vi "ReadConfigFile.vi"(1 "ConfigFilePath":path) -> (0 "Inst_parameters":T1)   [LabVIEW 2013]
uses:
  <vilib>/addons/h5labview2/file/H5Fmode.ctl
  <vilib>/addons/h5labview2/base/lib_path.vi
  <vilib>/addons/h5labview2/base/H5Equery.vi
  <vilib>/addons/h5labview2/attrib/H5Aread.llb/H5Aread.xnode
  <vilib>/addons/h5labview2/base/hid_t.ctl
  <vilib>/addons/h5labview2/file/H5F.lvlib
panel:
  out "Inst_list":string[](array[string])
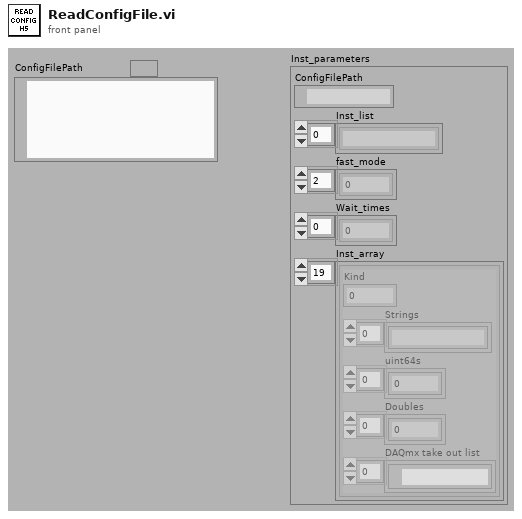
[diagram p1: front panel]
types:
  T1 = cluster{"ConfigFilePath":path, "Inst_list":string[], "fast_mode":u64[], "Wait_times":u64[], "Inst_array":cluster{"Kind":u16, "Strings":string[], "uint64s":u64[], "Doubles":dbl[], "DAQmx take out list":refnum<k21>[]}[]}
  T2 = cluster{"ConfigFilePath":path, "Inst_list":string[], "fast_mode":u16[], "Wait_times":u64[], "Inst_array":cluster{"Kind":u16, "Strings":string[], "uint16s":u64[], "Doubles":dbl[], refnum<k21>[]}[]}
  T3 = typedef "H5F.lvlib/H5Fmode.ctl" = enum16{"read-only", "read-write", "overwrite", "create new", "open or create"}
  T4 = cluster{"Kind":u16, "Strings":string[], "uint16s":u64[], "Doubles":dbl[], refnum<k21>[]}
  T5 = typedef "hid_t.ctl" = i32
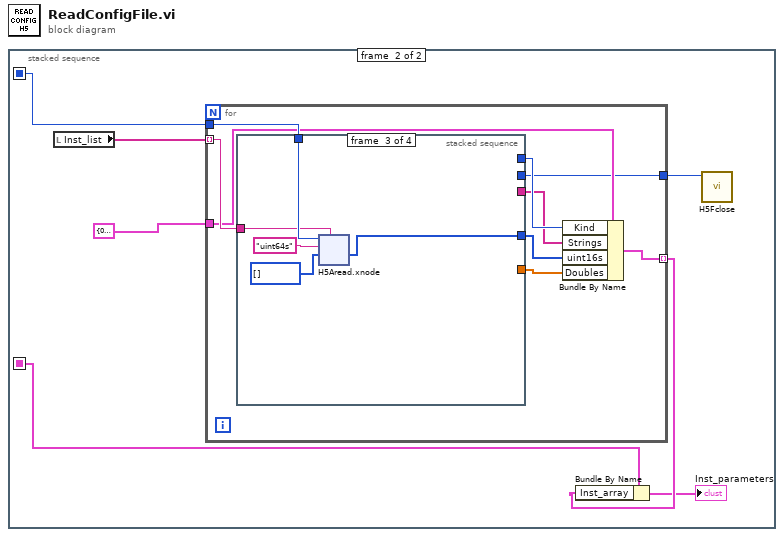
[diagram p0: block diagram]
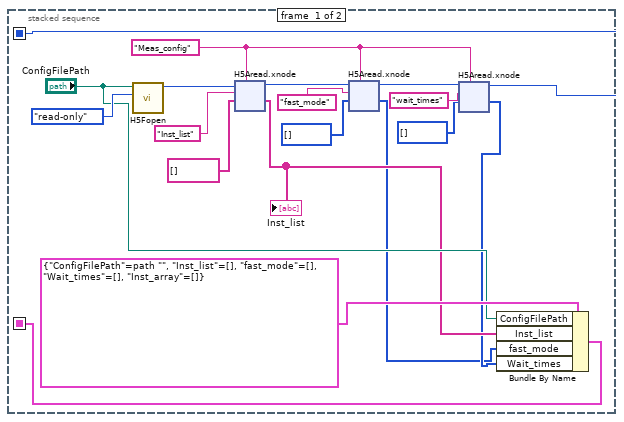
[diagram p2: hidden frame]
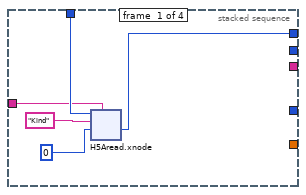
[diagram p3: hidden frame]
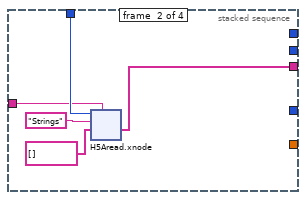
[diagram p4: hidden frame]
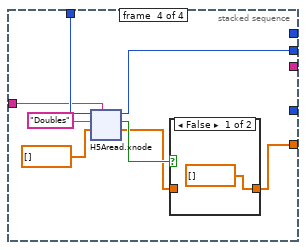
[diagram p5: hidden frame]
diagram:
  n1 = stacked-sequence {
    seq-local: [w1 _] -> [_ w69]
    seq-local: [w3 _] -> [_ w66]
    frame #0 {
      w9 = "Meas_config"
      n2 = call <vilib>:"H5Fopen.vi"("mode (read-only)"=H5Fmode."read-only" ("mode"), "path"="ConfigFilePath") -> ("ref out"=w16:T5)  [unwired: 8 in, 1 out]
      n3 = xnode "H5Aread.xnode"("object name"=w9, "default"=string[] [], "attrib name"="Inst_list", "ref in"=w16) -> ("data"=w5:string[], "ref out"=w14:T5)  [unwired: 2 in, 2 out]
      "Inst_list" <- w5
      n4 = xnode "H5Aread.xnode"("object name"=w9, "default"=u16[] [], "attrib name"="fast_mode", "ref in"=w14) -> ("data"=w2:u16[], "ref out"=w12:T5)  [unwired: 2 in, 2 out]
      n5 = xnode "H5Aread.xnode"("object name"=w9, "default"=u64[] [], "attrib name"="wait_times", "ref in"=w12) -> ("data"=w4:u64[], "ref out"=w1:T5)  [unwired: 2 in, 2 out]
      n6 = Bundle By Name(cluster=T2 {"ConfigFilePath"=path "", "Inst_list"=[], "fast_mode"=[], "Wait_times"=[], "Inst_array"=[]}, "ConfigFilePath"="ConfigFilePath", "Inst_list"=w5, "fast_mode"=w2, "Wait_times"=w4) -> (w3:T2)
    }
    frame #1 {
      n7 = local read "Inst_list"() -> (w70:string[])
      n8 = for {
        tunnel: w70 -> [w79] mode=indexing
        tunnel: w69 -> [w78]
        tunnel: T4 {"Kind"=0, "Strings"=[], "uint16s"=[], "Doubles"=[], []} -> [w76]
        tunnel: [w72] -> w65 mode=indexing
        tunnel: [w71] -> w67
        n9 = stacked-sequence {
          tunnel: w79 -> [w80 w100 w120 w140]
          tunnel: w78 -> [w83 w103 w123 w146]
          tunnel: [w81 _ _ _] -> w77
          tunnel: [_ w101 _ _] -> w75
          tunnel: [_ _ w121 _] -> w74
          tunnel: [_ _ _ w142] -> w73
          tunnel: [_ _ _ w141] -> w71
          frame #0 {
            n10 = xnode "H5Aread.xnode"("object name"=w80, "default"=u16 0, "attrib name"="Kind", "ref in"=w83) -> ("data"=w81:u16)  [unwired: 2 in, 3 out]
          }
          frame #1 {
            n11 = xnode "H5Aread.xnode"("object name"=w100, "default"=string[] [], "attrib name"="Strings", "ref in"=w103) -> ("data"=w101:string[])  [unwired: 2 in, 3 out]
          }
          frame #2 {
            n12 = xnode "H5Aread.xnode"("object name"=w120, "default"=u64[] [], "attrib name"="uint64s", "ref in"=w123) -> ("data"=w121:u64[])  [unwired: 2 in, 3 out]
          }
          frame #3 {
            n13 = xnode "H5Aread.xnode"("object name"=w140, "default"=dbl[] [], "attrib name"="Doubles", "ref in"=w146) -> ("data"=w143:dbl[], "found?"=w144:bool, "ref out"=w141:T5)  [unwired: 2 in, 1 out]
            n14 = case shown="False" w144 {
              tunnel: w143 -> [_ w149]
              tunnel: [dbl[] [] w149] -> w142
              frame False {
              }
              frame True {
              }
            }
          }
        }
        n15 = Bundle By Name(cluster=w76, "Kind"=w77, "Strings"=w75, "uint16s"=w74, "Doubles"=w73) -> (w72:T4)
      }
      n16 = Bundle By Name(cluster=w66, "Inst_array"=w65) -> (→"Inst_parameters":T2)
      n17 = call <vilib>:"H5Fclose.vi"("ref"=w67) -> ()  [unwired: 10 in, 1 out]
    }
  }
